vi "Load Config File.vi"(11 "In Cluster":T1) -> (3 "Out Cluster":T1)   [LabVIEW 2015]
uses:
  Typedef/Main Cluster.ctl
  Typedef/JSONCluster.ctl
  Typedef/Zone Data.ctl
  Typedef/Config JSON.ctl
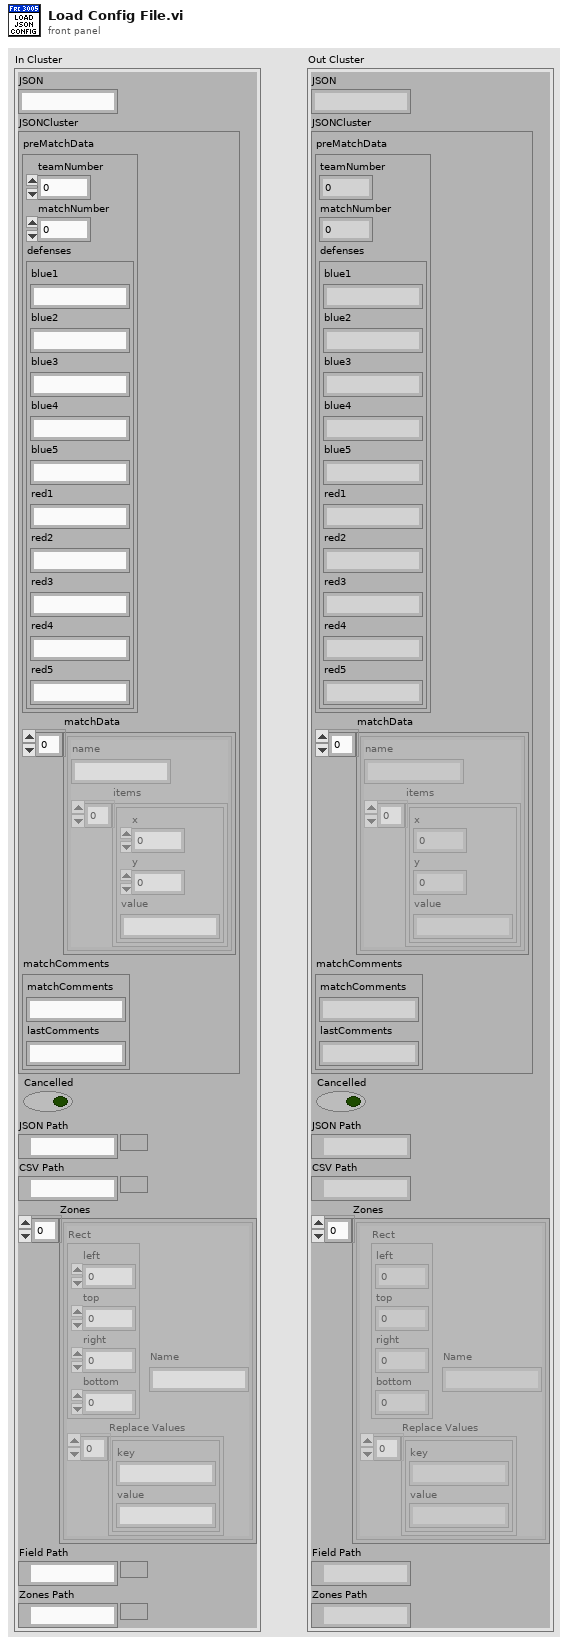
[diagram p1: front panel]
types:
  T1 = typedef "Main Cluster.ctl" = cluster{"JSON":string, "JSONCluster":T2, "Cancelled":bool, "JSON Path":path, "CSV Path":path, "Zones":T3[], "Field Path":path, "Zones Path":path}
  T2 = typedef "JSONCluster.ctl" = cluster{"preMatchData":cluster{"teamNumber":i32, "matchNumber":i32, "defenses":cluster{"blue1":string, "blue2":string, "blue3":string, "blue4":string, "blue5":string, "red1":string, "red2":string, "red3":string, "red4":string, "red5":string}}, "matchData":cluster{"name":string, "items":cluster{"x":i32, "y":i32, "value":string}[]}[], "matchComments":cluster{"matchComments":string, "lastComments":string}}
  T3 = typedef "Zone Data.ctl" = cluster{"Rect":cluster{"left":i16, "top":i16, "right":i16, "bottom":i16}, "Replace Values":cluster{"key":string, "value":string}[], "Name":string}
  T4 = typedef "Config JSON.ctl" = cluster{"Match JSON Path":string, "CSV Output Path":string, "Zone JSON Path":string}
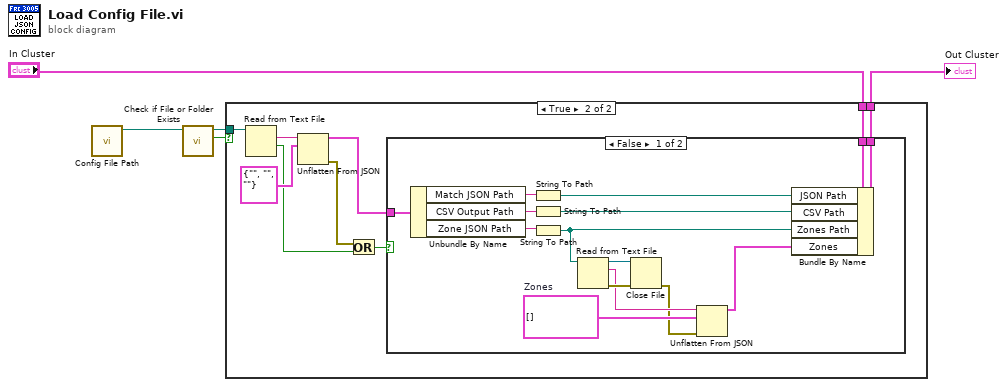
[diagram p0: block diagram]
diagram:
  n1 = call "Config File Path.vi"() -> ("appended path"=w3:path)  [unwired: 11 in]
  n2 = call <vilib>:"Check if File or Folder Exists.vi"("path"=w3) -> ("file or folder exists?"=w4:bool, "dup path"=w5:path)  [unwired: 8 in, 1 out]
  n3 = case shown="True" w4 {
    tunnel: w5 -> [_ w15]
    tunnel: "In Cluster" -> [w6 w8]
    tunnel: [w6 w7] -> w1
    frame False {
    }
    frame True {
      n4 = Read from Text File(file (use dialog)=w15) -> (text=w14:string, cancelled=w12:bool)  [unwired: 3 in, 2 out]
      n5 = Unflatten From JSON(JSON string=w14, type and defaults=T4 {"Match JSON Path"="", "CSV Output Path"="", "Zone JSON Path"=""}) -> (value=w9:T4, error out=w11:errorcluster)  [unwired: 5 in]
      n6 = Or(x=w11, y=w12) -> (x .or. y?=w10:bool)
      n7 = case shown="False" w10 {
        tunnel: w9 -> [w30 _]
        tunnel: w8 -> [w29 w31]
        tunnel: [w28 w31] -> w7
        frame False {
          w22 = T3[] []  # Zones
          n8 = Unbundle By Name(w30) -> ("Match JSON Path"=w25:string, "CSV Output Path"=w27:string, "Zone JSON Path"=w26:string)
          n9 = String To Path(string=w25) -> (path=w24:path)
          n10 = String To Path(string=w27) -> (path=w23:path)
          n11 = String To Path(string=w26) -> (path=w17:path)
          n12 = Read from Text File(file (use dialog)=w17) -> (refnum out=w20:refnum<file>, text=w19:string, error out=w21:errorcluster)  [unwired: 3 in, 1 out]
          n13 = Close File(refnum=w20, error in=w21) -> (error out=w18:errorcluster)  [unwired: 1 out]
          n14 = Unflatten From JSON(JSON string=w19, type and defaults=w22, error in (no error)=w18) -> (value=w16:T3[])  [unwired: 4 in, 1 out]
          n15 = Bundle By Name(cluster=w29, "JSON Path"=w24, "CSV Path"=w23, "Zones Path"=w17, "Zones"=w16) -> (w28:T1)
        }
        frame True {
        }
      }
    }
  }
  "Out Cluster" <- w1
